vi "Plural s.vi"(1 "# Elements":i32) -> (0 "Plural s":string)   [LabVIEW 2021, in "Strings.lvlib"]
uses:
  Strings.lvlib
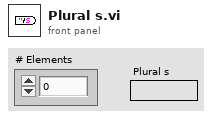
[diagram p1: front panel]
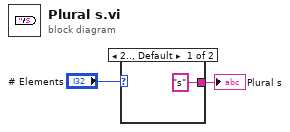
[diagram p0: block diagram]
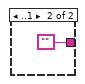
[diagram p2: hidden frame]
diagram:
  n1 = case shown="2.., Default" "# Elements" {
    tunnel: ["s" ""] -> w1
    frame 2.., Default {
    }
    frame ..1 {
    }
  }
  "Plural s" <- w1
